vi "qKET.vi"(0 "System no.":i32=1 min=1 max=4 step=1, 2 "Types to query":string[](array[string]), 5 "error in":errorcluster) -> (14 "Names":string[](array[string]), 19 "error out":errorcluster)   [LabVIEW 2026]
doc: "Returns active coordinate system types. The returned information depends on the arguments used. If no argument is set, all names of active coordinate systems are returned sorted by type.\n\nC-887, F-206, M-8X0: Only for GCS syntax version = GCS 2.0 or higher (Check with CSV?.vi. If CSV?.vi is not supported, syntax version is GCS 1.0)."
panel:
  # "Returns enabled coordinate system types. The returned information \ndepends on the arguments used."
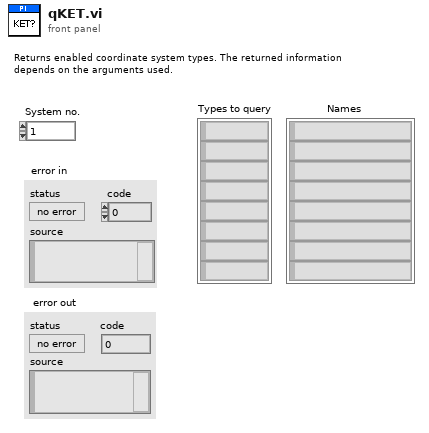
[diagram p1: front panel]
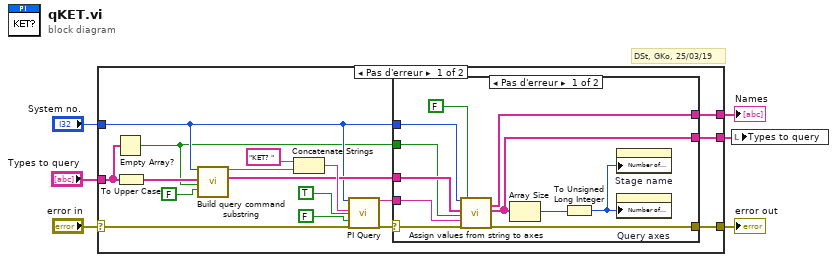
[diagram p0: block diagram]
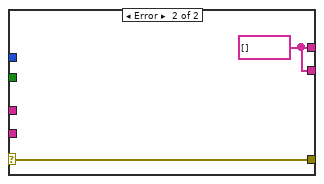
[diagram p2: hidden frame]
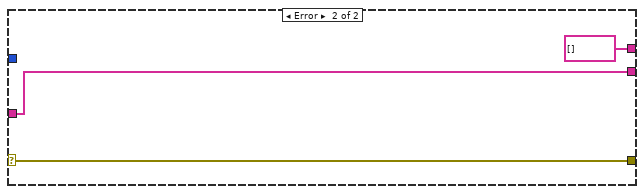
[diagram p3: hidden frame]
diagram:
  # "DSt, GKo, 25/03/19"
  n1 = case shown="Pas d'erreur" "error in" {
    selector: "error in" -> [w14 w38]
    tunnel: "Types to query" -> [w10 w37]
    tunnel: [w15 w38] -> w5
    tunnel: "System no." -> [w11 _]
    tunnel: [w17 string[] [] ("Strings")] -> w3
    tunnel: [w7 w37] -> w1
    frame No Error {
      n2 = Empty Array?(array=w10) -> (empty?=w9:bool)
      n3 = To Upper Case(1:w10) -> (0:w20:string[])
      n4 = call "Build query command substring.vi"("System no."=w11, "Axes to query in"=w20, "Query\nAll axes?"=w9, "For all axes: use\nAxis identifier?"=FALSE ("For all axes: use\nAxis identifier?")) -> ("Command substring"=w19:string, "Axes to query out"=w18:string[])  [unwired: 2 in, 12 out]
      n5 = Concatenate Strings("KET? ", w19) -> (w21:string)
      n6 = call "PI Query.vi"("System no."=w11, "String to send"=w21, "Attach termination char.?"=TRUE ("Attach Linefeed?"), "Strip spaces?"=FALSE, "error in"=w14) -> ("String read"=w12:string, "error out"=w8:errorcluster)  [unwired: 2 in, 11 out]
      n7 = case shown="Pas d'erreur" w8 {
        selector: w8 -> [w25 w36]
        tunnel: w18 -> [w34 _]
        tunnel: [w33 w35] -> w17
        tunnel: [w32 w36] -> w15
        tunnel: w12 -> [w29 _]
        tunnel: w11 -> [w27 _]
        tunnel: w9 -> [w26 _]
        tunnel: [w24 w35] -> w7
        frame No Error {
          n8 = call "Assign values from string to axes.vi"("System no."=w27, "Queried axes"=w34, "All axes queried?"=w26, "Input String"=w29, "error in"=w25, "Axes related?"=FALSE) -> ("Strings"=w33:string[], "Queried axes out"=w24:string[], "error out"=w32:errorcluster)  [unwired: 3 in, 8 out]
          n9 = Array Size(array=w24) -> (size(s)=w30:i32)
          n10 = To Unsigned Long Integer(number=w30) -> (unsigned 32bit integer=w28:u32)
          n11 = property on="Stage name" class="Tabl (strict)"("Number of Rows"=w28) -> ()  [unwired: 2 in, 2 out]
          n12 = property on="Query axes" class="Tabl (strict)"("Number of Rows"=w28) -> ()  [unwired: 2 in, 2 out]
        }
        frame Error {
          w35 = string[] [] ("Strings")
        }
      }
    }
    frame Error {
    }
  }
  "error out" <- w5
  "Names" <- w3
  n13 = local write "Types to query"(w1) -> ()
